vi "Secondary Heat Transfer Coefficient.vi"(4 "Thermal Conductivity of FLiNaK (W/m-K)":dbl, 6 "NDHX Tube Diameter (m)":dbl, 7 "Sec Pr":dbl, 9 "FLiNaK Viscosity (Pa-s)":dbl, 10 "FLiNaK Viscosity (Pa-s) 2":dbl, 11 "Sec Re":dbl) -> (3 "Sec Heat Xfer Coeff":dbl)   [LabVIEW 2019]
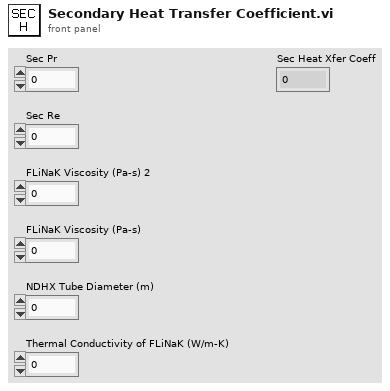
[diagram p1: front panel]
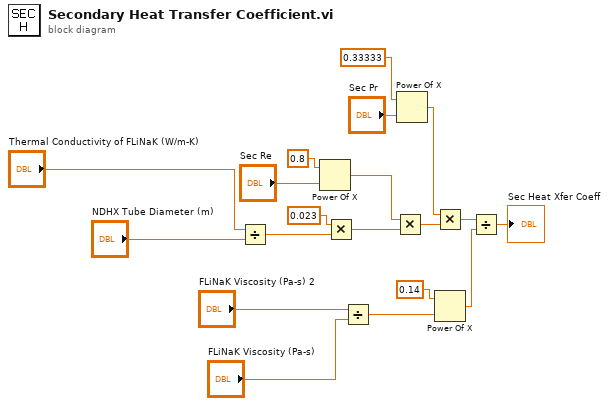
[diagram p0: block diagram]
diagram:
  n1 = Divide(x="Thermal Conductivity of FLiNaK (W/m-K)", y="NDHX Tube Diameter (m)") -> (x/y=w3:dbl)
  n2 = Power Of X(1:"Sec Re", 2:0.8 ("y")) -> (0:w8:dbl)
  n3 = Multiply(x=0.023, y=w3) -> (x*y=w5:dbl)
  n4 = Divide(x="FLiNaK Viscosity (Pa-s) 2", y="FLiNaK Viscosity (Pa-s)") -> (x/y=w15:dbl)
  n5 = Multiply(x=w8, y=w5) -> (x*y=w9:dbl)
  n6 = Power Of X(1:"Sec Pr", 2:0.33333 ("y")) -> (0:w12:dbl)
  n7 = Multiply(x=w12, y=w9) -> (x*y=w17:dbl)
  n8 = Power Of X(1:w15, 2:0.14 ("y")) -> (0:w18:dbl)
  n9 = Divide(x=w17, y=w18) -> (x/y=→"Sec Heat Xfer Coeff":dbl)
